vi "PTScanner.sync data to value.vi"(1 "byteArray":T2, 4 "nomValue":dbl, 9 "obj params":T1) -> (16 "matched":bool, 18 "actValue":dbl)   [LabVIEW 2014, in "PTScanner.lvlib"]
uses:
  PTScanner.lvlib
  CS_Core/CSSystem/CoreDefs/CoreDefs.rawDataType.ctl
  PTScanner.obj parameters.ctl
  CS_Core/CSSystem/CoreLib/CoreLib.byte array 2 string.vi
  CS_Core/CSSystem/CoreLib/CoreLib.byte array 2 double.vi
  CS_Core/CSSystem/CoreLib/CoreLib.byte array 2 float.vi
  CS_Core/CSSystem/CoreLib/CoreLib.byte array 2 int.vi
  CS_Core/CSSystem/CoreLib/CoreLib.byte array 2 short.vi
  CS_Core/CSSystem/CoreLib/CoreLib.lvlib
  _common/PTUtils/PTUtils.lvlib
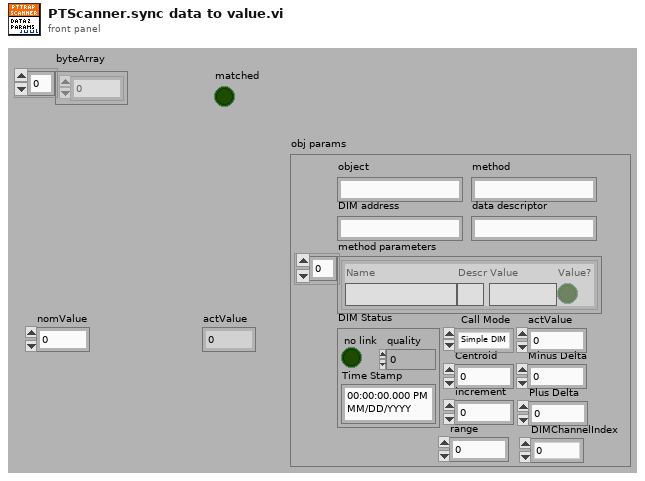
[diagram p1: front panel]
types:
  T1 = typedef "PTScanner.lvlib/PTScanner.obj parameters.ctl" = cluster{"object":string, "DIM address":string, "method":string, "data descriptor":string, "method parameters":cluster{"Name":string, "Descr":string, "Value":string, "Value?":bool}[], "Call Mode":enum16{"Simple DIM", "Synchronous"}, "actValue":dbl, "Centroid":dbl, "Minus Delta":dbl, "Plus Delta":dbl, "increment":dbl, "DIM Status":cluster{"no link":bool, "quality":i32, "Time Stamp":timestamp}, "range":dbl, "DIMChannelIndex":i32}
  T2 = typedef "CoreDefs.rawDataType.ctl" = i8[]
  T3 = cluster{"Name":string, "Descr":string, "Value":string, "Value?":bool}[]
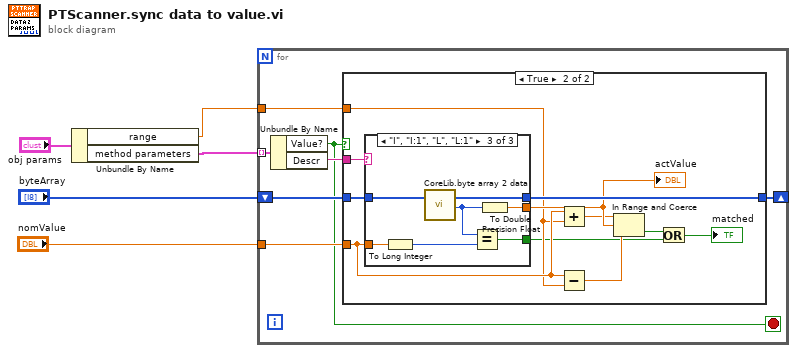
[diagram p0: block diagram]
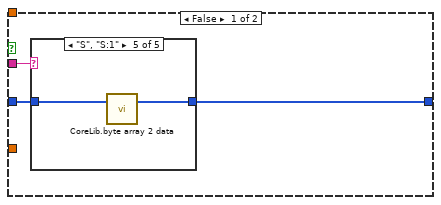
[diagram p2: hidden frame]
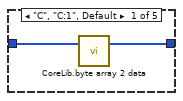
[diagram p3: hidden frame]
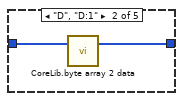
[diagram p4: hidden frame]
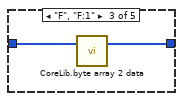
[diagram p5: hidden frame]
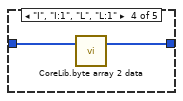
[diagram p6: hidden frame]
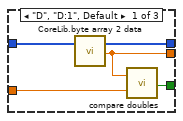
[diagram p7: hidden frame]
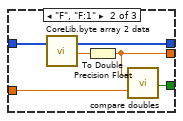
[diagram p8: hidden frame]
diagram:
  n1 = Unbundle By Name("obj params") -> ("range"=w1:dbl, "method parameters"=w2:T3)
  n2 = for {
    tunnel: w2 -> [w12] mode=indexing
    shift-right: [w10] -> _
    shift-left: "byteArray" -> [w9]
    tunnel: "nomValue" -> [w8]
    tunnel: w1 -> [w6]
    stop <- w7 stop-if-true
    n3 = Unbundle By Name(w12) -> ("Value?"=w7:bool, "Descr"=w11:string)
    n4 = case shown="True" w7 {
      tunnel: w11 -> [w15 w36]
      tunnel: [w14 w35] -> w10
      tunnel: w9 -> [w13 w34]
      tunnel: w8 -> [_ w32]
      tunnel: w6 -> [_ w31]
      frame False {
        n5 = case shown="\"S\", \"S:1\"" w15 {
          tunnel: [w16 w18 w20 w22 w24] -> w14
          tunnel: w13 -> [w17 w19 w21 w23 w25]
          frame "C", "C:1", Default {
            n6 = call-poly "CoreLib.byte array 2 data.vi"("byteArray"=w17) -> ("byteArray out"=w16:T2)  [unwired: 16 in, 2 out]
          }
          frame "D", "D:1" {
            n7 = call-poly "CoreLib.byte array 2 data.vi"("byteArray"=w19) -> ("byteArray out"=w18:T2)  [unwired: 16 in, 2 out]
          }
          frame "F", "F:1" {
            n8 = call-poly "CoreLib.byte array 2 data.vi"("byteArray"=w21) -> ("byteArray out"=w20:T2)  [unwired: 16 in, 2 out]
          }
          frame "I", "I:1", "L", "L:1" {
            n9 = call-poly "CoreLib.byte array 2 data.vi"("byteArray"=w23) -> ("byteArray out"=w22:T2)  [unwired: 16 in, 2 out]
          }
          frame "S", "S:1" {
            n10 = call-poly "CoreLib.byte array 2 data.vi"("byteArray"=w25) -> ("byteArray out"=w24:T2)  [unwired: 16 in, 2 out]
          }
        }
      }
      frame True {
        n11 = case shown="\"I\", \"I:1\", \"L\", \"L:1\"" w36 {
          tunnel: [w40 w46 w52] -> w35
          tunnel: w34 -> [w41 w47 w53]
          tunnel: w32 -> [w39 w45 w54]
          tunnel: [w38 w43 w50] -> w27
          tunnel: [w37 w42 w48] -> w33
          frame "D", "D:1", Default {
            n12 = call-poly "CoreLib.byte array 2 data.vi"("byteArray"=w41) -> ("byteArray out"=w40:T2, "d64"=w37:dbl)  [unwired: 16 in, 1 out]
            n13 = call "compare doubles.vi"("base value"=w37, "value to compare"=w39) -> ("Equal"=w38:bool)  [unwired: 17 in]
          }
          frame "F", "F:1" {
            n14 = call-poly "CoreLib.byte array 2 data.vi"("byteArray"=w47) -> ("byteArray out"=w46:T2, "f32"=w44:sgl)  [unwired: 16 in, 1 out]
            n15 = To Double Precision Float(number=w44) -> (double precision float=w42:dbl)
            n16 = call "compare doubles.vi"("base value"=w42, "value to compare"=w45) -> ("Equal"=w43:bool)  [unwired: 17 in]
          }
          frame "I", "I:1", "L", "L:1" {
            n17 = To Long Integer(number=w54) -> (32bit integer=w51:i32)
            n18 = call-poly "CoreLib.byte array 2 data.vi"("byteArray"=w53) -> ("byteArray out"=w52:T2, "i32"=w49:i32)  [unwired: 16 in, 1 out]
            n19 = Equal?(x=w49, y=w51) -> (x = y?=w50:bool)
            n20 = To Double Precision Float(number=w49) -> (double precision float=w48:dbl)
          }
        }
        "actValue" <- w33
        n21 = Add(x=w32, y=w31) -> (x+y=w30:dbl)
        n22 = Subtract(x=w32, y=w31) -> (x-y=w29:dbl)
        n23 = In Range and Coerce(upper limit=w30, x=w33, lower limit=w29) -> (In Range?=w28:bool)  [unwired: 1 out]
        n24 = Or(x=w28, y=w27) -> (x .or. y?=→"matched":bool)
      }
    }
  }
